vi "Write.vi"(10 "String":string, 11 "String in":refnum<class "String.lvclass">) -> (3 "String out":refnum<class "String.lvclass">)   [LabVIEW 2020, in "Data.lvlib" / "String.lvclass"]
doc: "Write string."
uses:
  String.lvclass
  String.lvclass/String.ctl
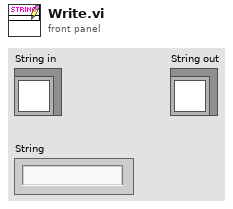
[diagram p1: front panel]
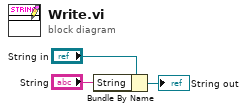
[diagram p0: block diagram]
diagram:
  n1 = Bundle By Name(cluster="String in", "String"="String") -> (→"String out":refnum<class "String.lvclass">)
